vi "Missing libraries on LV project.vi"(8 "error in (no error)":errorcluster, 11 "Path":path) -> (0 "error out":errorcluster, 3 "Pass":bool)   [LabVIEW 2021]
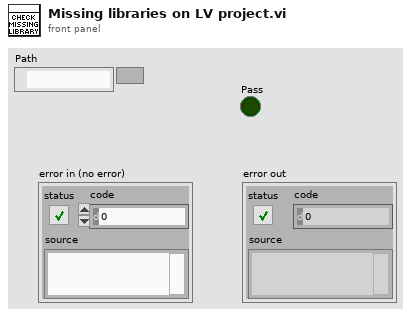
[diagram p1: front panel]
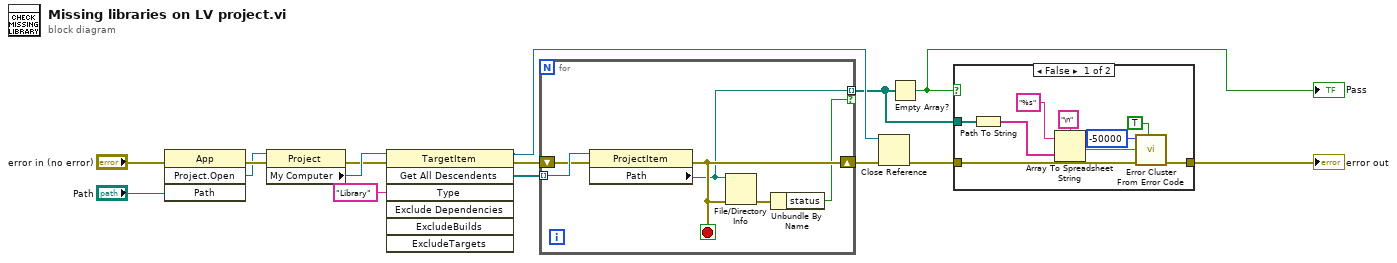
[diagram p0: block diagram]
diagram:
  n1 = invoke class="App" method="Project.Open"(error in="error in (no error)", "Path"="Path") -> (error out=w8:errorcluster, "Project:Open"=w6:refnum<vi>)  [unwired: 2 in, 2 out]
  n2 = property class="Project"(reference=w6, error in=w8) -> (error out=w12:errorcluster, "My Computer"=w15:refnum<vi>)  [unwired: 1 out]
  n3 = invoke class="TargetItem" method="Get All Descendents"(reference=w15, error in=w12, "Type"="Library") -> (reference out=w9:refnum<vi>, error out=w11:errorcluster, "All Descendents"=w13:refnum<vi>[])  [unwired: 4 in, 4 out]
  n4 = for {
    tunnel: w13 -> [w21] mode=indexing
    shift-right: [w18] -> w10
    shift-left: w11 -> [w20]
    tunnel: [w17] -> w1 mode=indexing if=w16
    stop <- w18 stop-if-true
    n5 = property class="ProjectItem"(reference=w21, error in=w20) -> (error out=w18:errorcluster, "Path"=w17:path)  [unwired: 1 out]
    n6 = File/Directory Info(path=w17, error in=w18) -> (error out=w19:errorcluster)  [unwired: 6 out]
    n7 = Unbundle By Name(w19) -> ("status"=w16:bool)
  }
  n8 = Close Reference(reference=w9, error in (no error)=w10) -> (error out=w4:errorcluster)
  n9 = Empty Array?(array=w1) -> (empty?=w3:bool)
  "Pass" <- w3
  n10 = case shown="False" w3 {
    tunnel: w1 -> [w29 _]
    tunnel: [w24 w31] -> w2
    tunnel: w4 -> [w23 w31]
    frame False {
      n11 = Path To String(path=w29) -> (string=w28:string[])
      n12 = Array To Spreadsheet String(delimiter (Tab)="\n", array=w28, 3:"%s" ("format string")) -> (spreadsheet string=w25:string)
      n13 = call <vilib>:"Error Cluster From Error Code.vi"("show call chain? (False)"=TRUE, "error in (no error)"=w23, "error message (\"\")"=w25, "error code (0)"=-50000) -> ("error out"=w24:errorcluster)  [unwired: 5 in]
    }
    frame True {
    }
  }
  "error out" <- w2
